vi "BRig_dataMTrig_warmup_cNoLick_R_reset.vi"() -> (2 "output_warmup_cNoLick_R_reset":i32)   [LabVIEW 2014]
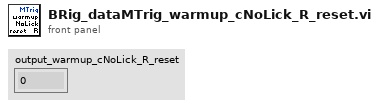
[diagram p1: front panel]
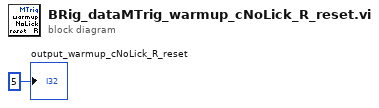
[diagram p0: block diagram]
diagram:
  "output_warmup_cNoLick_R_reset" <- 5 ("output_iBlock")
